vi "Create.vi"(9 "Actor Error":errorcluster, 10 "State":T1) -> (3 "Nested Status Message out":refnum<class "Nested Status Message.lvclass">)   [LabVIEW 2020, in "Artifex.lvlib" / "Nested Status Message.lvclass"]
uses:
  Nested Status Message.lvclass
  Actor State.ctl
  Nested Status Message.lvclass/Nested Status Message.ctl
  Artifex.lvlib
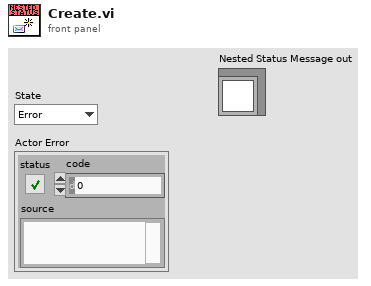
[diagram p1: front panel]
types:
  T1 = typedef "Artifex.lvlib/Actor State.ctl" = enum16{"Error", "Initialized", "Started", "Closing", "Closed"}
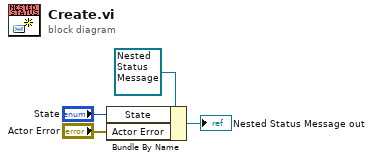
[diagram p0: block diagram]
diagram:
  n1 = Bundle By Name(cluster=refnum<class "Nested Status Message.lvclass"> refnum ("Nested Status Message in"), "State"="State", "Actor Error"="Actor Error") -> (→"Nested Status Message out":refnum<class "Nested Status Message.lvclass">)
